vi "Get_Indexes_of_Similar_Strigs.vi"(10 "Search":string, 11 "Input 1D array":string[](array[string])) -> (3 "Indexes":i32[](array[numeric]))   [LabVIEW 2022 SP3]
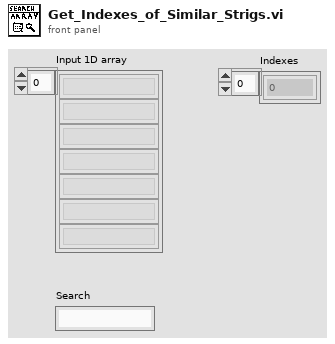
[diagram p1: front panel]
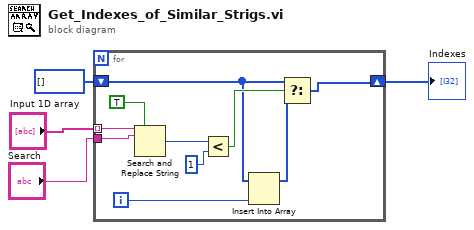
[diagram p0: block diagram]
diagram:
  n1 = for {
    shift-right: [w11] -> w2
    shift-left: i32[] [] -> [w5]
    tunnel: "Input 1D array" -> [w8] mode=indexing
    tunnel: "Search" -> [w7]
    i -> [w10]
    n2 = Search and Replace String(replace all?=TRUE ("replace all? (F)"), input string=w8, search string=w7) -> (number of replacements=w14:i32)  [unwired: 5 in, 3 out]
    n3 = Less?(x=w14, y=1) -> (x < y?=w12:bool)
    n4 = Insert Into Array(array=w5, new element=w10) -> (w9:i32[])  [unwired: 1 in]
    n5 = Select(t=w5, s=w12, f=w9) -> (s? t:f=w11:i32[])
  }
  "Indexes" <- w2
